vi "Start Measurements.vi"(6 "Reply to":refnum<class "Result Reply Msg.lvclass">, 7 "Objects enqueuers":refnum<class "Message Enqueuer.lvclass">[](array[class]), 8 "error in (no error)":errorcluster, 9 "Request type":T1, 10 "Objects":string[](array[string]), 11 "Pulse Controller in":refnum<class "Pulse Controller.lvclass">) -> (0 "error out":errorcluster, 3 "Pulse Controller out":refnum<class "Pulse Controller.lvclass">)   [LabVIEW 2018, in "Pulse Controller.lvclass"]
uses:
  Pulse Controller.lvclass
  C:/github/2018/LabActor/Worker/Worker.lvclass
  Template Module Messages/Result Reply Msg/Result Reply Msg.lvclass
  <vilib>/ActorFramework/Message Enqueuer/Message Enqueuer.lvclass
  Process Controller/Request type.ctl
  Worker/Worker.lvclass/Worker.ctl
  Pulse Controller.lvclass/Pulse Controller.ctl
  Template Module/Read State.vi
  Process Controller/Process Controller.lvclass
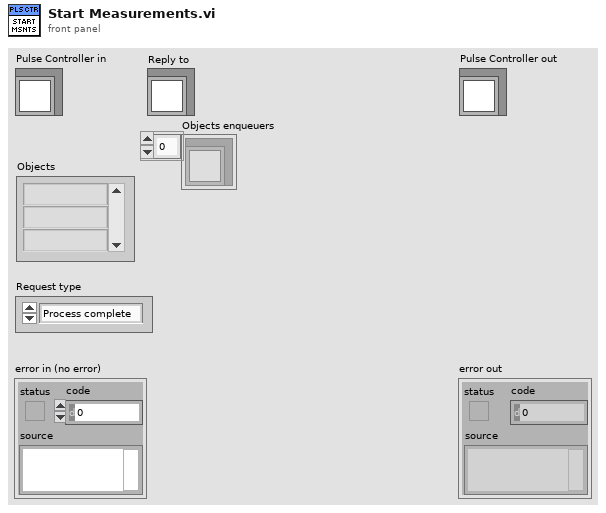
[diagram p1: front panel]
types:
  T1 = typedef "Request type.ctl" = enum16{"Process complete", "User command", "Auto-restart", "Error"}
  T2 = typedef "Worker State.ctl" = enum16{"Idle", "Starting", "Working", "Stopping"}
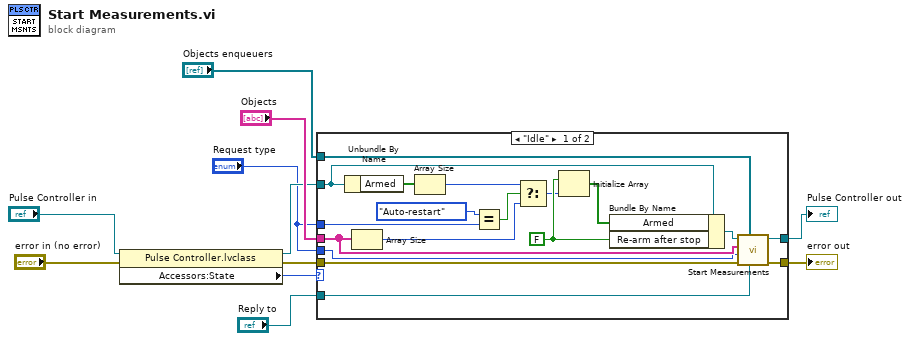
[diagram p0: block diagram]
diagram:
  n1 = property class="Pulse Controller.lvclass"(reference="Pulse Controller in", error in="error in (no error)") -> (reference out=w4:refnum<class "Pulse Controller.lvclass">, error out=w3:errorcluster, "Accessors:State"=w5:T2)
  n2 = case shown="\"Idle\"" w5 {
    tunnel: [w29 w31] -> w11
    tunnel: [w28 w30] -> w10
    tunnel: "Reply to" -> [w27 _]
    tunnel: "Objects enqueuers" -> [w26 _]
    tunnel: w3 -> [w25 w31]
    tunnel: "Objects" -> [w23 _]
    tunnel: w4 -> [w17 w30]
    tunnel: "Request type" -> [w20 _]
    tunnel: "Request type" -> [w19 _]
    frame "Idle" {
      w21 = FALSE
      n3 = Unbundle By Name(w17) -> ("Armed"=w16:bool[])
      n4 = Array Size(array=w23) -> (size(s)=w14:i32)
      n5 = Array Size(array=w16) -> (size(s)=w13:i32)
      n6 = Equal?(x=Request_type."Auto-restart", y=w19) -> (x = y?=w15:bool)
      n7 = Select(t=w13, s=w15, f=w14) -> (s? t:f=w12:i32)
      n8 = Initialize Array(w21, w12) -> (w22:bool[])
      n9 = Bundle By Name(cluster=w17, "Armed"=w22, "Re-arm after stop"=w21) -> (w24:refnum<class "Pulse Controller.lvclass">)
      n10 = call-parent "Start Measurements.vi"("Reply to"=w27, "Objects enqueuers"=w26, "error in (no error)"=w25, "Request type"=w20, "Objects"=w23, "Measure Controller in"=w24) -> ("error out"=w29:errorcluster, "Measure Controller out"=w28:refnum<class "Pulse Controller.lvclass">)  [unwired: 4 in]
    }
    frame "Working", Default {
    }
  }
  "error out" <- w11
  "Pulse Controller out" <- w10
